vi "Optiscan Test.vi"() -> ()   [LabVIEW 2012]
uses:
  <vilib>/Instr/_visa.llb/VISA Configure Serial Port (Instr).vi
panel:
  in  "write buffer":string="VERSION"
  out "read buffer":string
  # "G,0,0,0 = go absolute\nGR,0,0,0 = go relative\nP = Get position\n= = Limit switch status"
  # "Y axis buggered - limit switch stuck?"
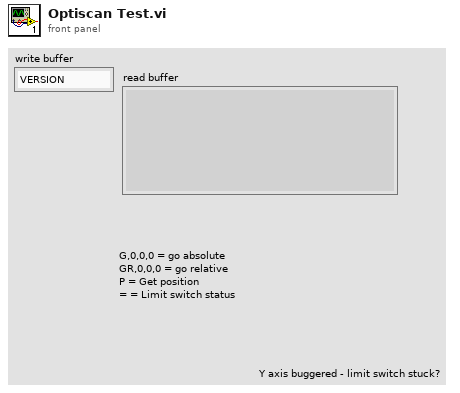
[diagram p1: front panel]
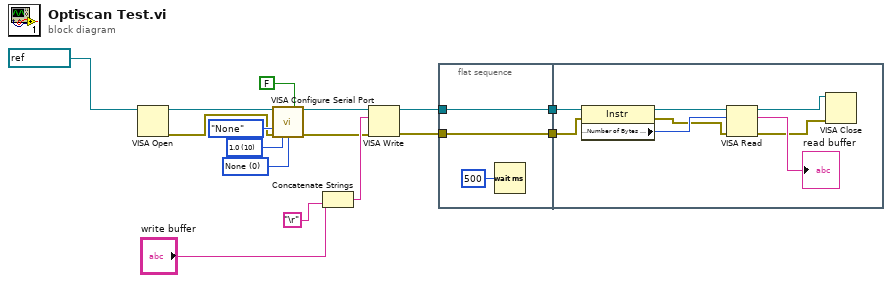
[diagram p0: block diagram]
diagram:
  w9 = u16 0 items=["None", "XON/XOFF", "RTS/CTS", "XON/XOFF & RTS/CTS", "DTR/DSR", "XON/XOFF & DTR/DSR"] ("flow control (0:none)")
  w10 = u16 10 items=["1.0"=10, "1.5"=15, "2.0"=20] ("stop bits (10: 1 bit)")
  n1 = VISA Open(VISA resource name=refnum<visa-resource-name> "COM3") -> (VISA resource name=w13:refnum<visa-resource-name>, error out=w4:errorcluster)  [unwired: 4 in]
  n2 = call-poly "VISA Configure Serial Port"("VISA resource name"=w13, "Enable Termination\nChar (T)"=FALSE ("Enable Termination\nChar (T)"), "parity (0:none)"=enum16{"None", "Odd", "Even", "Mark", "Space"}."None", "error in (no error)"=w4, "stop bits (10: 1 bit)"=w10, "flow control (0:none)"=w9) -> ("VISA resource name out"=w8:refnum<visa-resource-name>, "error out"=w5:errorcluster)  [unwired: 8 in]
  n3 = Concatenate Strings("write buffer", "\r") -> (w6:string)
  n4 = VISA Write(VISA resource name=w8, write buffer=w6, error in (no error)=w5) -> (VISA resource name out=w2:refnum<visa-resource-name>, error out=w3:errorcluster)  [unwired: 1 out]
  n5 = flat-sequence {
    tunnel: [w18] -> w16
    tunnel: w3 -> [w18]
    tunnel: [w17] -> w15
    tunnel: w2 -> [w17]
    tunnel: w16 -> [w26]
    tunnel: w15 -> [w27]
    frame #0 {
      n6 = Wait (ms)(milliseconds to wait=u32 500) -> ()  [unwired: 1 out]
    }
    frame #1 {
      n7 = property class="Instr"(reference=w27, error in=w26) -> (reference out=w24:refnum<visa-resource-name>, error out=w21:errorcluster, "Serial Settings:Number of Bytes at Serial Port"=w25:u32)
      n8 = VISA Read(VISA resource name=w24, byte count=w25, error in (no error)=w21) -> (VISA resource name out=w22:refnum<visa-resource-name>, read buffer=→"read buffer":string, error out=w20:errorcluster)  [unwired: 1 out]
      n9 = VISA Close(VISA resource name=w22, error in (no error)=w20) -> ()  [unwired: 1 out]
    }
  }
